vi "Update App.vi"(8 "error in (no error)":errorcluster, 10 "ViaApp":refnum<class "ViaApp.lvclass">, 11 "AppListPanel in":refnum<class "AppListPanel.lvclass">) -> (0 "error out":errorcluster, 3 "AppListPanel out":refnum<class "AppListPanel.lvclass">)   [LabVIEW 2020, in "PicoG-App.lvlib" / "AppListPanel.lvclass"]
uses:
  AppListPanel.lvclass
  ViaApp/ViaApp.lvclass
  AppListPanel.lvclass/AppListPanel.ctl
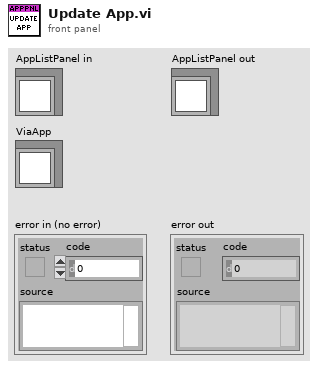
[diagram p1: front panel]
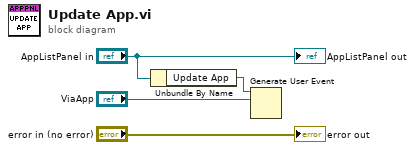
[diagram p0: block diagram]
diagram:
  n1 = Unbundle By Name("AppListPanel in") -> ("Update App"=w2:refnum<user-event>)
  n2 = Generate User Event(user event=w2, event data cluster="ViaApp") -> ()  [unwired: 2 in, 2 out]
  "error out" <- "error in (no error)"
  "AppListPanel out" <- "AppListPanel in"
